vi "Bulk Create.vi"(6 "commandTimeout":i32, 8 "error in (no error)":errorcluster, 9 "DynamicParameters":refnum<class "DynamicParameters.lvclass">[](array[class]), 10 "tableName":string, 11 "SqlMapper in":refnum<class "SqlMapper.lvclass">) -> (0 "error out":errorcluster, 2 "id":variant[](array[variant]), 3 "SqlMapper out":refnum<class "SqlMapper.lvclass">)   [LabVIEW 2020, in "ORM.lvlib" / "SqlMapper.lvclass"]
uses:
  SqlMapper.lvclass
  SqlMapper.lvclass/SqlMapper.ctl
  Query Result/Query Result.lvclass
  DbConnection/DbConnection.lvclass
  DynamicParameters/DynamicParameters.lvclass
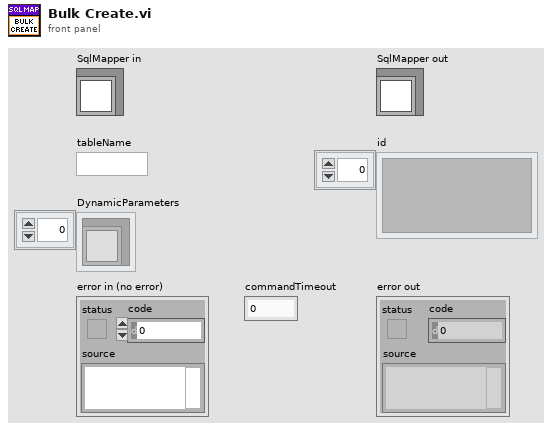
[diagram p1: front panel]
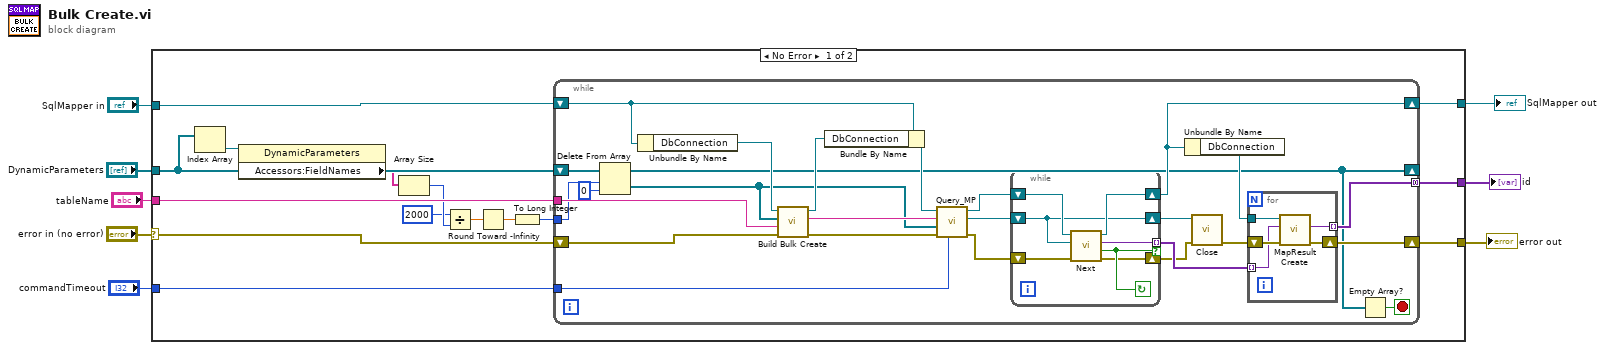
[diagram p0: block diagram]
diagram:
  n1 = case shown="No Error" "error in (no error)" {
    selector: "error in (no error)" -> [w23 w62]
    tunnel: "SqlMapper in" -> [w18 w63]
    tunnel: [w17 w63] -> w6
    tunnel: "DynamicParameters" -> [w16 _]
    tunnel: [w22 _] -> w4
    tunnel: [w21 w62] -> w3
    tunnel: "commandTimeout" -> [w19 _]
    tunnel: "tableName" -> [w20 _]
    frame No Error {
      n2 = Index Array(array=w16) -> (element=w15:refnum<class "DynamicParameters.lvclass">)  [unwired: 1 in]
      n3 = property class="DynamicParameters"(reference=w15) -> ("Accessors:FieldNames"=w14:string[])  [unwired: 1 in, 2 out]
      n4 = Array Size(array=w14) -> (size(s)=w13:i32)
      n5 = Divide(x=2000, y=w13) -> (x/y=w11:dbl)
      n6 = Round Toward -Infinity(1:w11) -> (0:w10:dbl)
      n7 = To Long Integer(number=w10) -> (32bit integer=w9:i32)
      n8 = while {
        tunnel: [w47] -> w22 mode=concatenating
        tunnel: w20 -> [w45]
        tunnel: w19 -> [w44]
        shift-right: [w46] -> w21
        shift-left: w23 -> [w49]
        shift-right: [w33] -> w17
        shift-left: w18 -> [w42]
        shift-right: [w24] -> _
        shift-left: w16 -> [w29]
        tunnel: w9 -> [w27]
        stop <- w25 stop-if-true
        n9 = Delete From Array(array=w29, length=w27, index=0) -> (deleted portion=w28:refnum<class "DynamicParameters.lvclass">[], array with subset deleted=w24:refnum<class "DynamicParameters.lvclass">[])
        n10 = Unbundle By Name(w42) -> ("DbConnection"=w48:refnum<class "DbConnection.lvclass">)
        n11 = call-dynamic "Build Bulk Create.vi"("error in (no error)"=w49, "tableName"=w45, "DynamicParameters in"=w28, "DbConnection in"=w48) -> ("error out"=w40:errorcluster, "BulkInsertQuery"=w35:string, "DbConnection out"=w43:refnum<class "DbConnection.lvclass">)  [unwired: 5 in]
        n12 = Bundle By Name(cluster=w42, "DbConnection"=w43) -> (w41:refnum<class "SqlMapper.lvclass">)
        n13 = call-dynamic "Query_MP.vi"("commandTimeout"=w44, "error in (no error)"=w40, "DynamicParameters"=w28, "sql"=w35, "SqlMapper in"=w41) -> ("error out"=w36:errorcluster, "Query Result out"=w39:refnum<class "Query Result.lvclass">, "SqlMapper out"=w37:refnum<class "SqlMapper.lvclass">)  [unwired: 4 in]
        n14 = while {
          shift-right: [w54] -> w32
          shift-left: w39 -> [w54]
          shift-right: [w55] -> w33
          shift-left: w37 -> [w56]
          tunnel: [w53] -> w34 mode=indexing if=w52
          shift-right: [w50] -> w31
          shift-left: w36 -> [w51]
          stop <- w52 continue-if-true
          n15 = call "Next.vi"("error in (no error)"=w51, "Query in"=w54, "SqlMapper in"=w56) -> ("error out"=w50:errorcluster, "found?"=w52:bool, "Row"=w53:variant, "SqlMapper out"=w55:refnum<class "SqlMapper.lvclass">)  [unwired: 5 in]
        }
        n16 = Unbundle By Name(w33) -> ("DbConnection"=w38:refnum<class "DbConnection.lvclass">)
        n17 = call-dynamic "Close.vi"("error in (no error)"=w31, "Query Result in"=w32) -> ("error out"=w30:errorcluster)  [unwired: 9 in]
        n18 = for {
          tunnel: [w61] -> w47 mode=indexing
          tunnel: w38 -> [w59]
          shift-right: [w60] -> w46
          shift-left: w30 -> [w58]
          tunnel: w34 -> [w57] mode=indexing
          n19 = call-dynamic "MapResult Create.vi"("error in (no error)"=w58, "InsertResultVariant"=w57, "DbConnection in"=w59) -> ("error out"=w60:errorcluster, "ID"=w61:variant)  [unwired: 7 in]
        }
        n20 = Empty Array?(array=w24) -> (empty?=w25:bool)
      }
    }
    frame Error {
    }
  }
  "error out" <- w3
  "SqlMapper out" <- w6
  "id" <- w4
